vi "Config.vi"(8 "error in (no error)":errorcluster, 10 "Setting":variant, 11 "NI Fgen in":refnum<class "NI Fgen.lvclass">) -> (0 "error out":errorcluster, 3 "NI Fgen out":refnum<class "NI Fgen.lvclass">)   [LabVIEW 2025, in "Fgen.lvlib" / "NI Fgen.lvclass"]
uses:
  NI Fgen.lvclass
  NI Fgen.lvclass/NI Fgen.ctl
  <instrlib>/niFgen/niFgen.llb/niFgen Trigger Mode.ctl
  Fgen configuration/Fgen configuration.lvclass
  <instrlib>/niFgen/niFgen.llb/niFgen Output Impedance.ctl
  Fgen Channel/Fgen Channel.lvclass
  Fgen Channel configuration/Fgen Channel configuration.lvclass
  <instrlib>/niFgen/niFgen.llb/niFgen Configure Software Edge Start Trigger.vi
  <instrlib>/niFgen/niFgen.llb/niFgen Create Waveform (DBL).vi
  <instrlib>/niFgen/niFgen.llb/niFgen Disable Start Trigger.vi
  <instrlib>/niFgen/niFgen.llb/niFgen Configure Digital Edge Start Trigger.vi
  Users/Public/Documents/Sandia National Labs/TSS Plugin/Abstract Engine.lvlibp/Abstract Instrument/Channel.ctl
  Users/Public/Documents/Sandia National Labs/TSS Plugin/Abstract Engine.lvlibp/Abstract Instrument/Abstract Instrument.lvclass
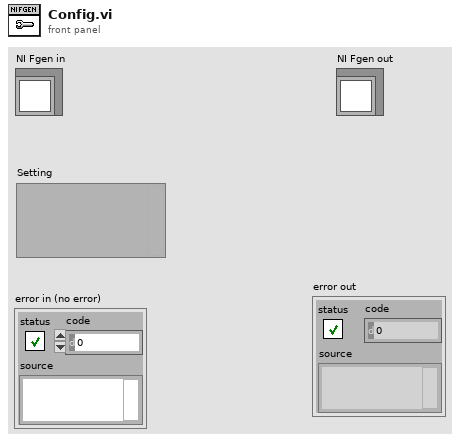
[diagram p1: front panel]
types:
  T1 = typedef "Abstract Engine.lvlibp/Instrument configuration.lvclass/Default Instrument.ctl" = cluster{"Type":string, "Address":string, "SW Alias":string, "Description":string, "Enabled":bool}
  T2 = typedef "Fgen.lvlib/Fgen configuration.lvclass/Fgen Setting.ctl" = cluster{"Type":string, "Output Mode":string, "Sample Rate":dbl, "Samples":dbl, "Gain":dbl, "Trigger":string, "Impedance":string, "Offset":dbl}
  T3 = cluster{"Waveform Type":u16, "Amplitude":dbl, "# of points":u32}[]
  T4 = typedef "Abstract Engine.lvlibp/Abstract Instrument.lvclass/Channel.ctl" = cluster{"Alias":string, "DataType":enum16{"Anaolg Input", "Waveform"}, "Unit":enum16{"---", "V", "A", "Ohm", "Hz", "uF", "degC", "deg"}, "Upper limit":dbl, "Lower limit":dbl, "Measurement":variant}
  T5 = typedef "niFgen Output Impedance.ctl" = i32
  T6 = typedef "niFgen Trigger Mode.ctl" = i32
  T7 = typedef "Fgen.lvlib/Fgen Channel configuration.lvclass/Fgen Channel Setting.ctl" = cluster{"Trgger Type":string, "Duty Cycle":dbl, "Amplitude":dbl, "Frequency":dbl, "Output Shape":string, "Phase":dbl}
  T8 = typedef "Abstract Engine.lvlibp/Channel configuration.lvclass/Default Channel.ctl" = cluster{"Address":string, "SW Alias":string, "Enabled":bool, "Type":string, "Description":string}
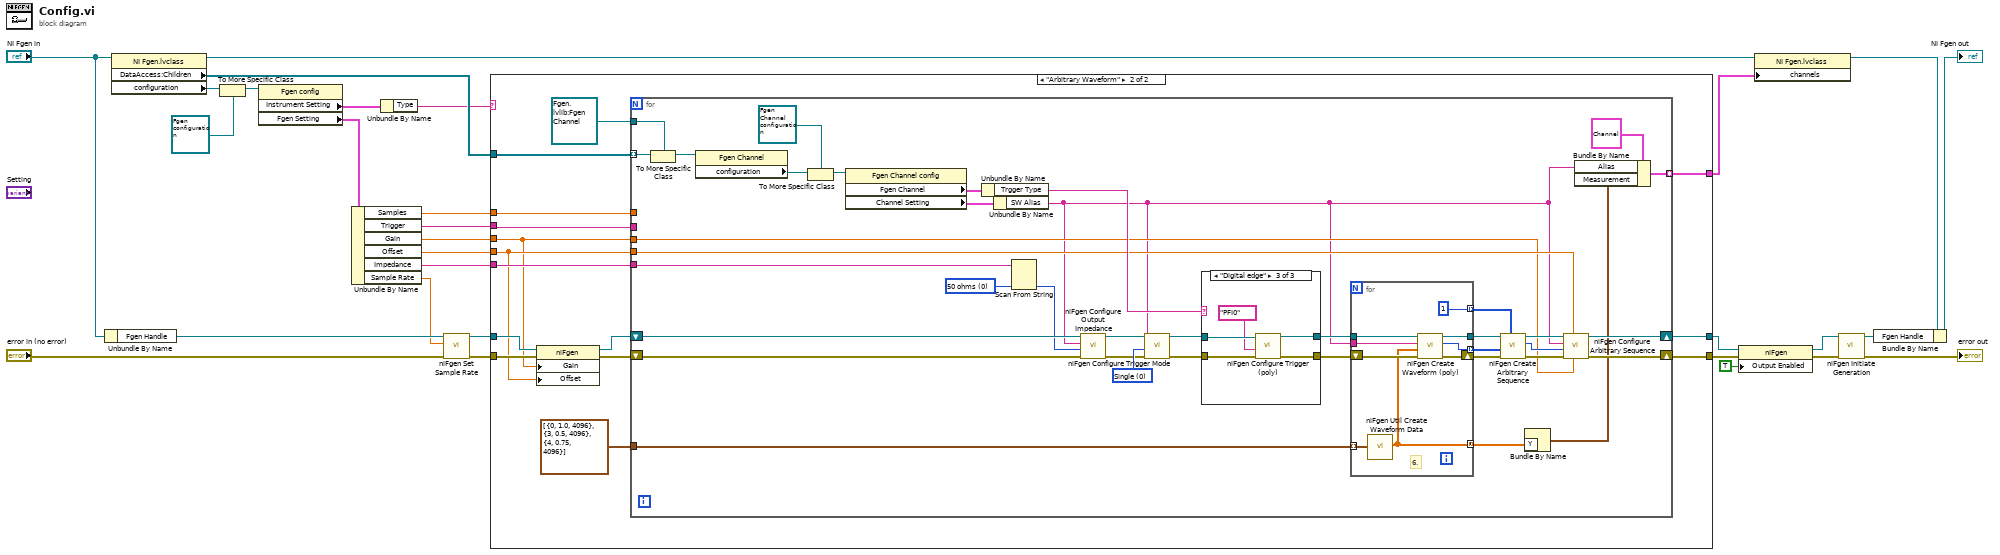
[diagram p0: block diagram]
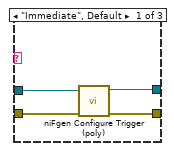
[diagram p3: hidden frame]
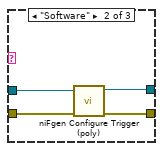
[diagram p4: hidden frame]
diagram:
  n1 = Unbundle By Name("NI Fgen in") -> ("Fgen Handle"=w22:refnum<k15>)
  n2 = property class="NI Fgen.lvclass"(reference="NI Fgen in") -> (reference out=w26:refnum<class "NI Fgen.lvclass">, "DataAccess:Children"=w16:refnum<data-value>[], "configuration"=w25:refnum<class "CEF_serializable configuration.lvclass">)  [unwired: 1 in, 1 out]
  n3 = To More Specific Class(target class=refnum<class "Fgen configuration.lvclass"> refnum ("Fgen.lvlib:Fgen configuration.lvclass"), reference=w25) -> (specific class reference=w23:refnum<class "Fgen configuration.lvclass">)  [unwired: 1 in, 1 out]
  n4 = property class="Fgen config"(reference=w23) -> ("Instrument Setting"=w4:T1, "Fgen Setting"=w2:T2)  [unwired: 1 in, 2 out]
  n5 = Unbundle By Name(w2) -> ("Samples"=w15:dbl, "Trigger"=w14:string, "Gain"=w17:dbl, "Offset"=w18:dbl, "Impedance"=w5:string, "Sample Rate"=w6:dbl)
  n6 = Unbundle By Name(w4) -> ("Type"=w3:string)
  n7 = call <instrlib>:"niFgen Set Sample Rate.vi"("error in (no error)"="error in (no error)", "Sample Rate (Samp/s)"=w6, "Instrument Handle"=w22) -> ("error out"=w20:errorcluster, "Instrument Handle Out"=w19:refnum<k15>)  [unwired: 7 in]
  n8 = case shown="\"Arbitrary Waveform\"" w3 {
    tunnel: w20 -> [w31 w46]
    tunnel: w19 -> [w30 w45]
    tunnel: w18 -> [_ w36]
    tunnel: w17 -> [_ w35]
    tunnel: w5 -> [_ w37]
    tunnel: w16 -> [_ w40]
    tunnel: w15 -> [_ w39]
    tunnel: w14 -> [_ w38]
    tunnel: [w30 w43] -> w9
    tunnel: [w31 w41] -> w13
    tunnel: [_ w32] -> w1
    frame "Standard Waveform", Default {
    }
    frame "Arbitrary Waveform" {
      n9 = property class="niFgen"(reference=w45, error in=w46, "Gain"=w35, "Offset"=w36) -> (reference out=w44:refnum<k15>, error out=w42:errorcluster)
      n10 = for {
        shift-right: [w67] -> w41
        shift-left: w42 -> [w81]
        shift-right: [w63] -> w43
        shift-left: w44 -> [w80]
        tunnel: w40 -> [w84] mode=indexing
        tunnel: refnum<data-value> refnum ("data value reference") -> [w83]
        tunnel: w39 -> [_]
        tunnel: w38 -> [_]
        tunnel: w37 -> [w58]
        tunnel: w36 -> [w62]
        tunnel: w35 -> [w61]
        tunnel: T3 [{"Waveform Type"=0, "Amplitude"=1.0, "# of points"=4096}, {"Waveform Type"=3, "Amplitude"=0.5, "# of points"=4096}, {"Waveform Type"=4, "Amplitude"=0.75, "# of points"=4096}] ("Waveform Array") -> [w60]
        tunnel: [w49] -> w32 mode=indexing
        w57 = T5 0 items=["50 ohms", "75 ohms"] ("Impedance (default: 0=50 ohms)")
        w79 = T6 0 items=["Single", "Continuous", "Stepped", "Burst"] ("Trigger Mode (default: 1=continuous)")
        n11 = To More Specific Class(target class=w83, reference=w84) -> (specific class reference=w82:refnum<data-value>)  [unwired: 1 in, 1 out]
        n12 = property class="Fgen Channel"(reference=w82) -> ("configuration"=w55:refnum<class "CEF_serializable configuration.lvclass">)  [unwired: 1 in, 2 out]
        n13 = To More Specific Class(target class=refnum<class "Fgen Channel configuration.lvclass"> refnum ("Fgen.lvlib:Fgen Channel config"), reference=w55) -> (specific class reference=w54:refnum<class "Fgen Channel configuration.lvclass">)  [unwired: 1 in, 1 out]
        n14 = property class="Fgen Channel config"(reference=w54) -> ("Fgen Channel"=w52:T7, "Channel Setting"=w51:T8)  [unwired: 1 in, 2 out]
        n15 = Unbundle By Name(w52) -> ("Trgger Type"=w75:string)
        n16 = Unbundle By Name(w51) -> ("SW Alias"=w50:string)
        n17 = Scan From String(input string=w58, default 1=w57) -> (output 1=w56:T5)  [unwired: 3 in, 3 out]
        n18 = call <instrlib>:"niFgen Configure Output Impedance.vi"("error in (no error)"=w81, "Impedance (default: 0=50 ohms)"=w56, "Channel Name"=w50, "Instrument Handle"=w80) -> ("error out"=w78:errorcluster, "Instrument Handle Out"=w77:refnum<k15>)  [unwired: 6 in]
        n19 = call <instrlib>:"niFgen Configure Trigger Mode.vi"("error in (no error)"=w78, "Trigger Mode (default: 1=continuous)"=w79, "Channel Name"=w50, "Instrument Handle"=w77) -> ("error out"=w76:errorcluster, "Instrument Handle Out"=w74:refnum<k15>)  [unwired: 6 in]
        n20 = case shown="\"Digital edge\"" w75 {
          tunnel: [w97 w101 w106] -> w72
          tunnel: w74 -> [w96 w100 w105]
          tunnel: w76 -> [w95 w99 w104]
          tunnel: [w94 w98 w103] -> w73
          frame "Immediate", Default {
            # "Single"
            n21 = call-poly <instrlib>:"niFgen Configure Trigger (poly).vi"("error in (no error)"=w95, "Instrument Handle"=w96) -> ("error out"=w94:errorcluster, "Instrument Handle Out"=w97:refnum<k15>)  [unwired: 8 in]
          }
          frame "Software" {
            # "Continuous"
            n22 = call-poly <instrlib>:"niFgen Configure Trigger (poly).vi"("error in (no error)"=w99, "Instrument Handle"=w100) -> ("error out"=w98:errorcluster, "Instrument Handle Out"=w101:refnum<k15>)  [unwired: 8 in]
          }
          frame "Digital edge" {
            # "Steps"
            n23 = call-poly <instrlib>:"niFgen Configure Trigger (poly).vi"("error in (no error)"=w104, "Source"="PFI0" ("Source (PFI 0)"), "Instrument Handle"=w105) -> ("error out"=w103:errorcluster, "Instrument Handle Out"=w106:refnum<k15>)  [unwired: 7 in]
          }
        }
        n24 = for {
          tunnel: [w93] -> w66
          tunnel: [w92] -> w64 mode=indexing
          shift-right: [w90] -> w68
          shift-left: w73 -> [w91]
          tunnel: [1] -> w65 mode=indexing
          tunnel: w72 -> [w88]
          tunnel: w60 -> [w87] mode=indexing
          tunnel: w50 -> [w86]
          tunnel: [w85] -> w59 mode=concatenating
          # "6."
          n25 = call <instrlib>:"niFgen Util Create Waveform Data.vi"("Waveform"=w87) -> ("Waveform Data"=w85:dbl[])  [unwired: 10 in]
          n26 = call-poly <instrlib>:"niFgen Create Waveform (poly).vi"("error in (no error)"=w91, "Waveform Data Array"=w85, "Channel Name"=w86, "Instrument Handle"=w88) -> ("error out"=w90:errorcluster, "Waveform Handle"=w92:i32, "Instrument Handle Out"=w93:refnum<k15>)  [unwired: 5 in]
        }
        n27 = call <instrlib>:"niFgen Create Arbitrary Sequence.vi"("Loop Counts Array"=w65, "error in (no error)"=w68, "Waveform Handles Array"=w64, "Instrument Handle"=w66) -> ("error out"=w70:errorcluster, "Sequence Handle"=w69:i32, "Instrument Handle Out"=w71:refnum<k15>)  [unwired: 5 in]
        n28 = Bundle By Name("Y"=w59) -> (w48:waveform(dbl))  [unwired: 1 in]
        n29 = call <instrlib>:"niFgen Configure Arbitrary Sequence.vi"("Gain"=w61, "Offset"=w62, "error in (no error)"=w70, "Sequence Handle"=w69, "Channel Name"=w50, "Instrument Handle"=w71) -> ("error out"=w67:errorcluster, "Instrument Handle Out"=w63:refnum<k15>)  [unwired: 4 in]
        n30 = Bundle By Name(cluster=T4 {"Alias"="ch0", "DataType"=enum."Anaolg Input", "Unit"=enum."V", "Upper limit"=10.0, "Lower limit"=-10.0, "Measurement"=variant} ("Channel"), "Alias"=w50, "Measurement"=w48) -> (w49:T4)
      }
    }
  }
  n31 = property class="niFgen"(reference=w9, error in=w13, "Output Enabled"=TRUE ("Output:Output Enabled")) -> (reference out=w8:refnum<k15>, error out=w10:errorcluster)
  n32 = property class="NI Fgen.lvclass"(reference=w26, "channels"=w1) -> (reference out=w28:refnum<class "NI Fgen.lvclass">)  [unwired: 1 in, 1 out]
  n33 = call <instrlib>:"niFgen Initiate Generation.vi"("error in (no error)"=w10, "Instrument Handle"=w8) -> ("error out"=→"error out":errorcluster, "Instrument Handle Out"=w11:refnum<k15>)  [unwired: 8 in]
  n34 = Bundle By Name(cluster=w28, "Fgen Handle"=w11) -> (→"NI Fgen out":refnum<class "NI Fgen.lvclass">)
